vi "Check 2D Limits_entwurf.vi"(2 "error in":T2, 3 "Magnitude Limit (kG)":dbl format="%.3f", 4 "Z-Axis Communications Config":T1={"GPIB address"=22, "GPIB bus"=0, "connection ID"=refnum, "IP"="192.168.2.200", "Active Comm Interface"=0, "Serial Port"="", "Programmer Type"=0} {"Programmer Type" items=["Model 430", "Model 420"]; "Active Comm Interface" items=["TCP/IP (Model 430 Only)", "RS232", "IEEE488"]}, 5 "Y-Axis Communications Config":T1={"GPIB address"=22, "GPIB bus"=0, "connection ID"=refnum, "IP"="192.168.2.200", "Active Comm Interface"=0, "Serial Port"="", "Programmer Type"=0} {"Programmer Type" items=["Model 430", "Model 420"]; "Active Comm Interface" items=["TCP/IP (Model 430 Only)", "RS232", "IEEE488"]}, 6 "Z-Axis Field (kG)":dbl format="%.3f", 7 "Y-Axis Field (kG)":dbl format="%.3f") -> (0 "Within Limits?":bool, 1 "error out":T2)   [LabVIEW 2009]
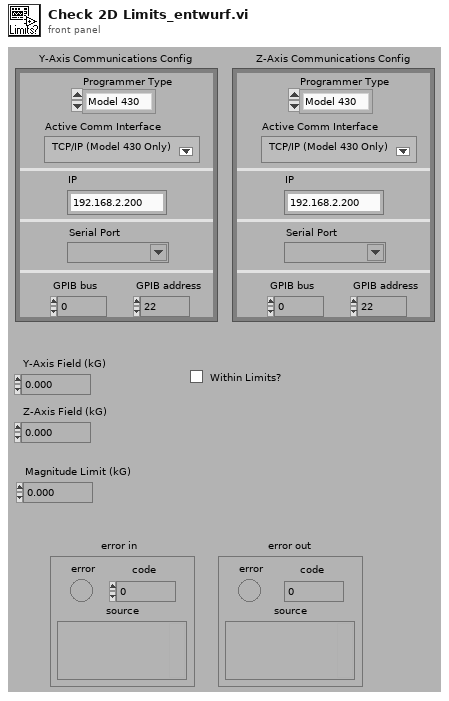
[diagram p1: front panel]
types:
  T1 = cluster{"GPIB address":i16, "GPIB bus":i16, "connection ID":refnum<k5>, "IP":string, "Active Comm Interface":u16, "Serial Port":refnum<visa-resource-name>, "Programmer Type":u16}
  T2 = cluster{"error":bool, "code":i32, "source":string}
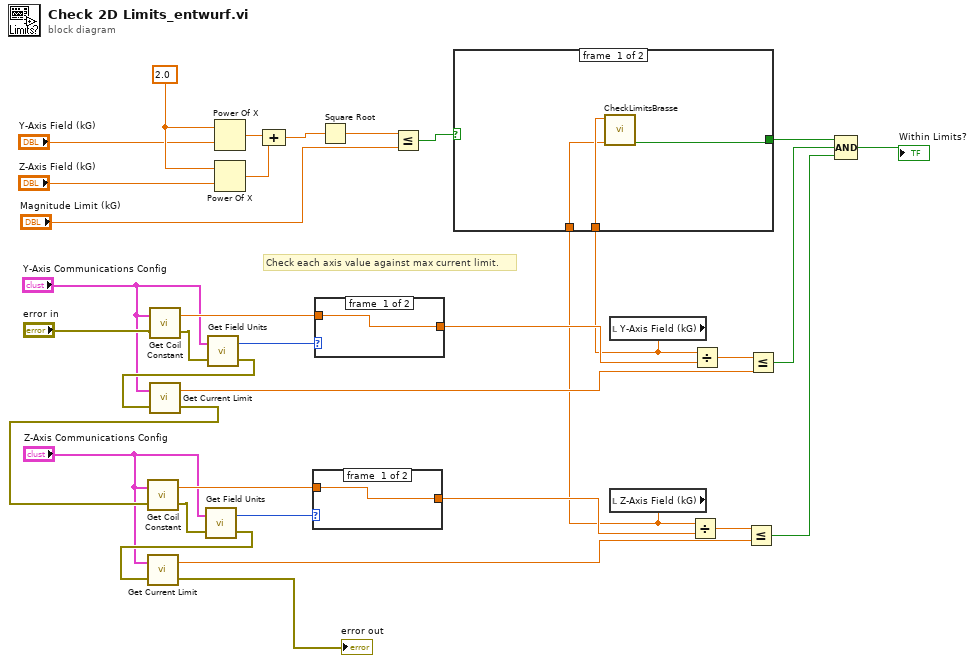
[diagram p0: block diagram]
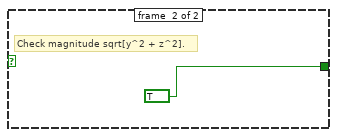
[diagram p2: hidden frame]
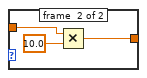
[diagram p3: hidden frame]
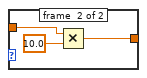
[diagram p4: hidden frame]
diagram:
  w34 = 2.0 ("x")
  # "Check each axis value against max current limit."
  n1 = call <userlib>:"Get Coil Constant.vi"("error in"="error in", "Communications Config"="Y-Axis Communications Config") -> ("error out"=w19:T2, "Coil Constant"=w20:dbl)
  n2 = call <userlib>:"Get Field Units.vi"("error in"=w19, "Communications Config"="Y-Axis Communications Config") -> ("error out"=w18:T2, "Field Units"=w21:enum16{"kg", "t"})
  n3 = call <userlib>:"Get Current Limit.vi"("error in"=w18, "Communications Config"="Y-Axis Communications Config") -> ("error out"=w13:T2, "Current Limit (A)"=w11:dbl)
  n4 = call <userlib>:"Get Coil Constant.vi"("error in"=w13, "Communications Config"="Z-Axis Communications Config") -> ("error out"=w15:T2, "Coil Constant"=w16:dbl)
  n5 = call <userlib>:"Get Field Units.vi"("error in"=w15, "Communications Config"="Z-Axis Communications Config") -> ("error out"=w14:T2, "Field Units"=w17:enum16{"kg", "t"})
  n6 = call <userlib>:"Get Current Limit.vi"("error in"=w14, "Communications Config"="Z-Axis Communications Config") -> ("error out"=→"error out":T2, "Current Limit (A)"=w9:dbl)
  n7 = Power Of X(1:"Y-Axis Field (kG)", 2:w34) -> (0:w31:dbl)
  n8 = Power Of X(1:"Z-Axis Field (kG)", 2:w34) -> (0:w30:dbl)
  n9 = Compound Arithmetic op=ADD(w31, w30) -> (w24:dbl)
  n10 = case shown="\"kg\", Default" w17 {
    tunnel: w16 -> [w35 w37]
    tunnel: [w35 w36] -> w10
    frame #0 {
    }
    frame #1 {
      n11 = Multiply(x=w37, y=10.0) -> (x*y=w36:dbl)
    }
  }
  n12 = case shown="\"t\"" w21 {
    tunnel: w20 -> [w39 w41]
    tunnel: [w39 w40] -> w12
    frame #0 {
    }
    frame #1 {
      n13 = Multiply(x=w41, y=10.0) -> (x*y=w40:dbl)
    }
  }
  n14 = Square Root(x=w24) -> (sqrt(x)=w23:dbl)
  n15 = Less Or Equal?(x=w23, y="Magnitude Limit (kG)") -> (x <= y?=w4:bool)
  n16 = local read "Y-Axis Field (kG)"() -> (w2:dbl)
  n17 = local read "Z-Axis Field (kG)"() -> (w1:dbl)
  n18 = case shown="True" w4 {
    tunnel: [w45 TRUE] -> w3
    tunnel: w2 -> [w44 _]
    tunnel: w1 -> [w43 _]
    frame #0 {
      n19 = call "CheckLimitsBrasse.vi"("Z-Axis Field (kG)"=w43, "Y-Axis Field (kG)"=w44) -> ("Within Limit"=w45:bool)  [unwired: 9 in]
    }
    frame #1 {
      # "Check magnitude sqrt[y^2 + z^2]."
    }
  }
  n20 = Divide(x=w1, y=w10) -> (x/y=w28:dbl)
  n21 = Divide(x=w2, y=w12) -> (x/y=w29:dbl)
  n22 = Less Or Equal?(x=w28, y=w9) -> (x <= y?=w26:bool)
  n23 = Less Or Equal?(x=w29, y=w11) -> (x <= y?=w27:bool)
  n24 = Compound Arithmetic op=AND(w3, w27, w26) -> (→"Within Limits?":bool)
